vi "_Write.vi"(8 "error in (no error)":errorcluster, 10 "data":string, 11 "file descriptor":u64) -> (0 "error out":errorcluster, 3 "written":i32)   [LabVIEW 2020, in "NI_Subprocess.lvlib" / "Subprocess.lvclass"]
doc: "Writes some (not necessarily all) <b>data</b> to the specified <b>file descriptor</b>. The operation is non-blocking."
uses:
  <vilib>/Subprocess/Subprocess/Subprocess.lvclass
  lviosrg.dll
  <vilib>/ErrorRing/Error Ring.xnode
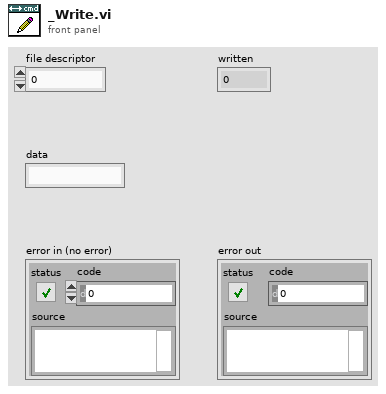
[diagram p1: front panel]
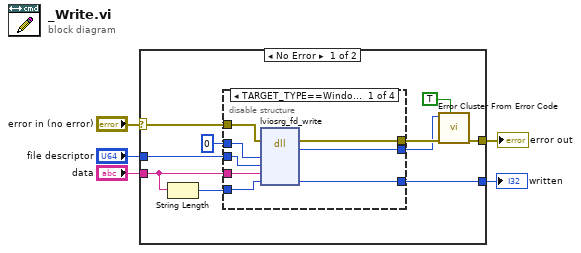
[diagram p0: block diagram]
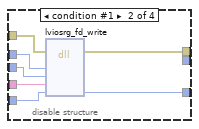
[diagram p2: hidden frame]
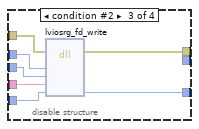
[diagram p3: hidden frame]
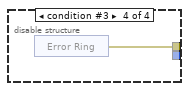
[diagram p4: hidden frame]
diagram:
  n1 = case shown="No Error" "error in (no error)" {
    selector: "error in (no error)" -> [w11 w43]
    tunnel: [w8 _] -> w5
    tunnel: "data" -> [w15 _]
    tunnel: "file descriptor" -> [w14 _]
    tunnel: [w7 w43] -> w2
    frame No Error {
      n2 = String Length(string=w15) -> (length=w13:i32)
      n3 = disable-structure shown="TARGET_TYPE==Windows||OS==Win" {
        disable-tunnel: [w23 w30 w37 _] -> w8
        disable-tunnel: [w22 w29 w36 w38] -> w9
        disable-tunnel: w15 -> [w21 w28 w35 _]
        disable-tunnel: w14 -> [w20 w27 w34 _]
        disable-tunnel: w13 -> [w19 w26 w33 _]
        disable-tunnel: 0 ("errno") -> [w18 w25 w32 _]
        disable-tunnel: w11 -> [w17 w24 w31 _]
        disable-tunnel: [w16 _ _ _] -> w6
        frame condition #0 (active) {
          n4 = dll-call lib="lviosrg.*" fn="lviosrg_fd_write"(error in=w17, "errno"=w18, "write_fd"=w20, "buf"=w21, "buflen"=w19) -> (error out=w22:errorcluster, "return type"=w16:i32, "buflen"=w23:i32)  [unwired: 5 in, 1 out]
        }
        frame condition #1 {
          n5 = dll-call lib="lviosrg.*" fn="lviosrg_fd_write"(error in=w24, "errno"=w25, "write_fd"=w27, "buf"=w28, "buflen"=w26) -> (error out=w29:errorcluster, "buflen"=w30:i32)  [unwired: 6 in, 1 out]
        }
        frame condition #2 {
          n6 = dll-call lib="lviosrg.*" fn="lviosrg_fd_write"(error in=w31, "errno"=w32, "write_fd"=w34, "buf"=w35, "buflen"=w33) -> (error out=w36:errorcluster, "buflen"=w37:i32)  [unwired: 6 in, 1 out]
        }
        frame condition #3 {
          n7 = xnode "Error Ring"() -> ("error out"=w38:errorcluster)
        }
      }
      n8 = call <vilib>:"Error Cluster From Error Code.vi"("show call chain? (False)"=TRUE, "error in (no error)"=w9, "error code (0)"=w6) -> ("error out"=w7:errorcluster)  [unwired: 6 in]
    }
    frame Error {
    }
  }
  "written" <- w5
  "error out" <- w2
